vi "PXI-Data Available Queue (1D).vi"(11 "error in (no error)":errorcluster) -> (6 "Waveform Graph":dbl[][](graph), 8 "Abort Send Data Queue":bool, 10 "AI Waveforms":dbl[](array[numeric]), 15 "error out":errorcluster)   [LabVIEW 2020]
uses:
  DAQ Engine VIs/PXI Globals.vi
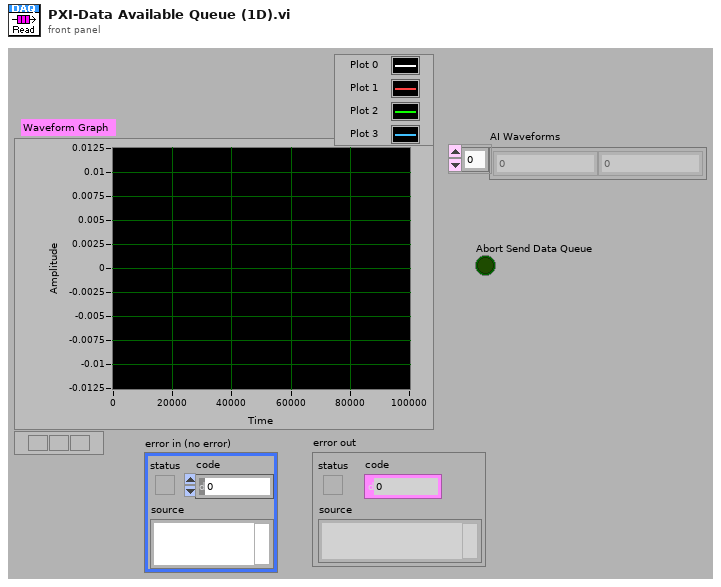
[diagram p1: front panel]
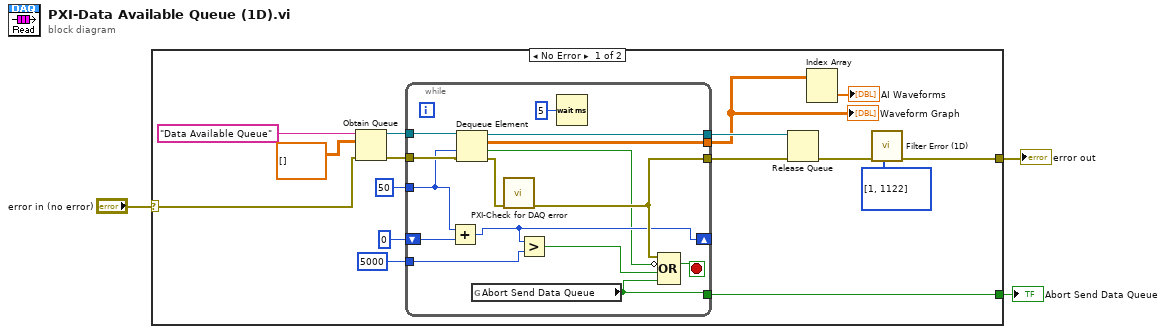
[diagram p0: block diagram]
diagram:
  n1 = case shown="No Error" "error in (no error)" {
    selector: "error in (no error)" -> [w15 w35]
    tunnel: [w10 w35] -> w3
    tunnel: [w6 _] -> w1
    frame No Error {
      n2 = Obtain Queue(name (unnamed)="Data Available Queue", element data type=dbl[][] [] ("AI Waveforms 2"), error in (no error)=w15) -> (queue out=w17:refnum<queue>, error out=w14:errorcluster)  [unwired: 2 in, 1 out]
      n3 = while {
        tunnel: [w27] -> w12
        tunnel: w17 -> [w34]
        tunnel: [w33] -> w4
        tunnel: [w32] -> w16
        tunnel: w14 -> [w29]
        tunnel: 50 ("timeout in ms (-1)") -> [w25]
        shift-right: [w24] -> _
        shift-left: 0 -> [w26]
        tunnel: 5000 ("timeout in ms (-1)") -> [w23]
        tunnel: [w20] -> w6
        stop <- w31 stop-if-true
        n4 = Add(x=w25, y=w26) -> (x+y=w24:i32)
        n5 = Dequeue Element(queue=w34, timeout in ms (-1)=w25, error in (no error)=w29) -> (queue out=w32:refnum<queue>, element=w33:dbl[][], timed out?=w21:bool, error out=w30:errorcluster)
        n6 = global read "PXI Globals.vi" "Abort Send Data Queue"() -> (w20:bool)
        n7 = call "PXI-Check for DAQ error.vi"("error in (no error)"=w30) -> ("error out"=w27:errorcluster)  [unwired: 14 in]
        n8 = Greater?(x=w24, y=w23) -> (0:w22:bool)
        n9 = Wait (ms)(milliseconds to wait=u32 5) -> ()  [unwired: 1 out]
        n10 = Compound Arithmetic op=OR(w27, invert w21, w22, w20) -> (w31:bool)
      }
      "Waveform Graph" <- w4
      n11 = Release Queue(queue=w16, error in (no error)=w12) -> (error out=w11:errorcluster)  [unwired: 1 in, 2 out]
      n12 = Index Array(array=w4) -> (element=→"AI Waveforms":dbl[])  [unwired: 2 in]
      n13 = call "Filter Error (1D).vi"("error in (no error)"=w11, "Array"=i32[] [1, 1122]) -> ("error out"=w10:errorcluster)  [unwired: 9 in]
    }
    frame Error {
    }
  }
  "error out" <- w3
  "Abort Send Data Queue" <- w1
